vi "Write Axis Position data.vi"(7 "Send any changes now? (F)":bool, 8 "error in (no error)":errorcluster, 10 "Current Position":dbl[unit], 11 "Fiber Auto Collimation state data in":refnum<class "Fiber Auto Collimation state data.lvclass">) -> (0 "error out":errorcluster, 3 "Fiber Auto Collimation state data out":refnum<class "Fiber Auto Collimation state data.lvclass">)   [LabVIEW 2018, in "Fiber Auto Collimation state data.lvclass"]
doc: "This \"LIV test data\" is just a placeholder and example for how real test data might be stored. This accessor plus its data in the state data class private control probably need to be removed or replaced with something to hold test data for the actual station."
uses:
  Fiber Auto Collimation state data.lvclass
  Fiber Auto Collimation state data.lvclass/Fiber Auto Collimation state data.ctl
  Tracked state data.ctl
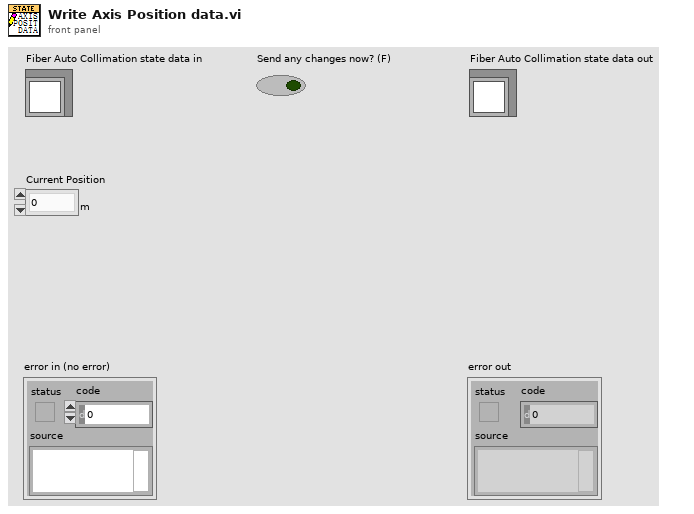
[diagram p1: front panel]
types:
  T1 = typedef "Fiber Auto Collimation state data.lvclass/Tracked state data.ctl" = enum16{"No update", "Permission level", "Username", "Test running", "DUT Serial", "Test status", "MOM Lot", "Loaded test recipe", "Model case running", "Station status", "BV data", "Defect Identify data", "Axis Position data", "Fiber Ass PN", "Operator", "RunTime", "VBAI", "Steps Cycle Time"}
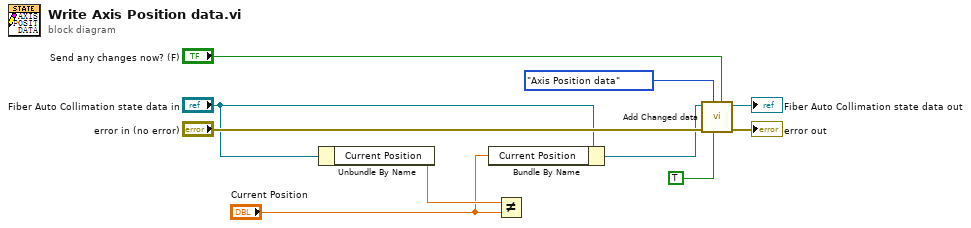
[diagram p0: block diagram]
diagram:
  n1 = Unbundle By Name("Fiber Auto Collimation state data in") -> ("Current Position"=w4:dbl[unit])
  n2 = Bundle By Name(cluster="Fiber Auto Collimation state data in", "Current Position"="Current Position") -> (w7:refnum<class "Fiber Auto Collimation state data.lvclass">)
  n3 = Not Equal?(x=w4, y="Current Position") -> ()  [unwired: 1 out]
  n4 = call "Add Changed data.vi"("Send any changes now? (F)"="Send any changes now? (F)", "Data changed?"=TRUE, "Data type"=Tracked_state_data."Axis Position data", "error in (no error)"="error in (no error)", "Fiber Auto Collimation state data in"=w7) -> ("error out"=→"error out":errorcluster, "Fiber Auto Collimation state data out"=→"Fiber Auto Collimation state data out":refnum<class "Fiber Auto Collimation state data.lvclass">)  [unwired: 5 in]
